vi "FormatDMAelement_8_elements.vi"(8 "valid in":bool, 11 "Data in":fxp<+/-,16,14>[](array[numeric])=[0.0, 0.0, 0.0, 0.0, 0.0, 0.0, 0.0, 0.0]) -> (0 "valid out":bool, 3 "Values":u64[](array[numeric]))   [LabVIEW 2018]
uses:
  <vilib>/rvi/FXPMathLib/FxpInterpret/XNode/nifxpmath_Interpret.xnode
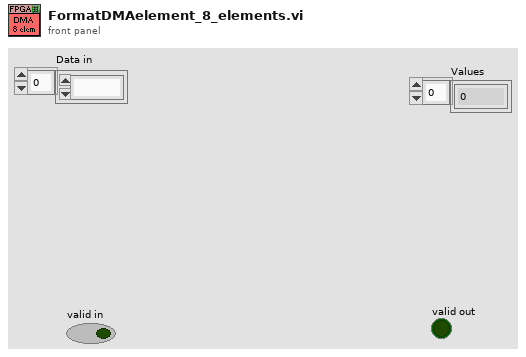
[diagram p1: front panel]
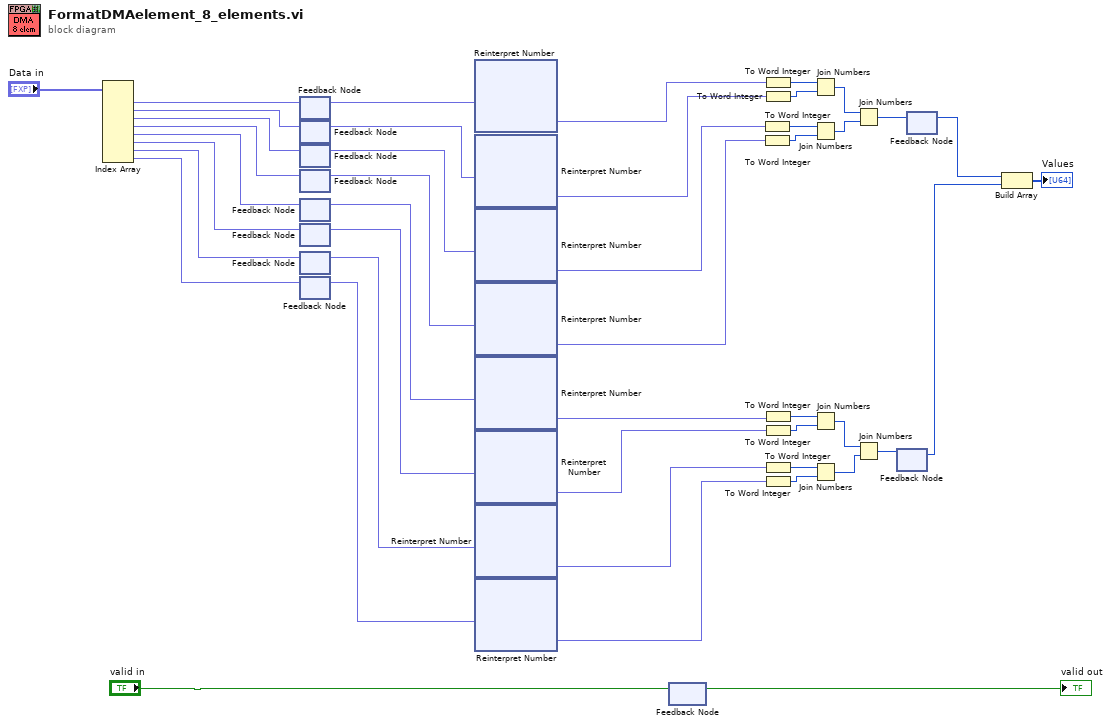
[diagram p0: block diagram]
diagram:
  n1 = Index Array(array="Data in") -> (element #1=w41:fxp<+/-,16,14>, element #2=w40:fxp<+/-,16,14>, element #3=w39:fxp<+/-,16,14>, element #4=w38:fxp<+/-,16,14>, element #5=w23:fxp<+/-,16,14>, element #6=w22:fxp<+/-,16,14>, element #7=w9:fxp<+/-,16,14>, element #8=w8:fxp<+/-,16,14>)  [unwired: 8 in]
  n2 = feedback #1() -> (w31:fxp<+/-,16,14>)  [unwired: 1 in]
  n3 = feedback-in #1(w41) -> ()
  n4 = feedback #2() -> (w29:fxp<+/-,16,14>)  [unwired: 1 in]
  n5 = feedback-in #2(w40) -> ()
  n6 = feedback #3() -> (w28:fxp<+/-,16,14>)  [unwired: 1 in]
  n7 = feedback-in #3(w39) -> ()
  n8 = feedback #4() -> (w27:fxp<+/-,16,14>)  [unwired: 1 in]
  n9 = feedback-in #4(w38) -> ()
  n10 = feedback #5() -> (w21:fxp<+/-,16,14>)  [unwired: 1 in]
  n11 = feedback-in #5(w23) -> ()
  n12 = feedback #6() -> (w20:fxp<+/-,16,14>)  [unwired: 1 in]
  n13 = feedback-in #6(w22) -> ()
  n14 = feedback #7() -> (w7:fxp<+/-,16,14>)  [unwired: 1 in]
  n15 = feedback-in #7(w9) -> ()
  n16 = feedback #8() -> (w6:fxp<+/-,16,14>)  [unwired: 1 in]
  n17 = feedback-in #8(w8) -> ()
  n18 = xnode "Reinterpret Number"("x"=w31) -> ("y"=w30:fxp<+/-,16,16>)
  n19 = xnode "Reinterpret Number"("x"=w29) -> ("y"=w26:fxp<+/-,16,16>)
  n20 = xnode "Reinterpret Number"("x"=w28) -> ("y"=w25:fxp<+/-,16,16>)
  n21 = xnode "Reinterpret Number"("x"=w27) -> ("y"=w24:fxp<+/-,16,16>)
  n22 = xnode "Reinterpret Number"("x"=w21) -> ("y"=w16:fxp<+/-,16,16>)
  n23 = xnode "Reinterpret Number"("x"=w20) -> ("y"=w15:fxp<+/-,16,16>)
  n24 = xnode "Reinterpret Number"("x"=w7) -> ("y"=w3:fxp<+/-,16,16>)
  n25 = xnode "Reinterpret Number"("x"=w6) -> ("y"=w2:fxp<+/-,16,16>)
  n26 = feedback #9() -> (→"valid out":bool)  [unwired: 1 in]
  n27 = feedback-in #9("valid in") -> ()
  n28 = To Word Integer(number=w25) -> (16bit integer=w35:i16)
  n29 = To Word Integer(number=w24) -> (16bit integer=w34:i16)
  n30 = To Word Integer(number=w30) -> (16bit integer=w36:i16)
  n31 = To Word Integer(number=w26) -> (16bit integer=w37:i16)
  n32 = To Word Integer(number=w16) -> (16bit integer=w18:i16)
  n33 = To Word Integer(number=w15) -> (16bit integer=w17:i16)
  n34 = To Word Integer(number=w3) -> (16bit integer=w4:i16)
  n35 = To Word Integer(number=w2) -> (16bit integer=w5:i16)
  n36 = Join Numbers(hi=w36, lo=w37) -> ((hi.lo)=w33:u32)
  n37 = Join Numbers(hi=w35, lo=w34) -> ((hi.lo)=w32:u32)
  n38 = Join Numbers(hi=w18, lo=w17) -> ((hi.lo)=w19:u32)
  n39 = Join Numbers(hi=w4, lo=w5) -> ((hi.lo)=w1:u32)
  n40 = Join Numbers(hi=w33, lo=w32) -> ((hi.lo)=w14:u64)
  n41 = Join Numbers(hi=w19, lo=w1) -> ((hi.lo)=w13:u64)
  n42 = feedback #10() -> (w12:u64)  [unwired: 1 in]
  n43 = feedback-in #10(w13) -> ()
  n44 = feedback #11() -> (w11:u64)  [unwired: 1 in]
  n45 = feedback-in #11(w14) -> ()
  n46 = Build Array(w11, w12) -> (→"Values":u64[])
